vi "test bindata forth and back v2.vi"() -> ()   [LabVIEW 2018, in "LV-Julia_ZMQ-Roundtrip_lib.lvlib"]
uses:
  LV-Julia_ZMQ-Roundtrip_lib.lvlib
  05036e79-a137-49d8-b8bd-98c2707dfc19.vi
  d20d9b8d-18a0-4bcc-837d-245d5138e077.vi
  42358c4e-b4d2-4416-9aa8-9e7cd75d6887.vi
  32c35eaf-297e-4906-af2c-c0a637e2c9ed.vi
  05036e79-a137-49d8-b8bd-98c2707dfc19.vi/b16ececd-46f8-40b8-a446-7cfb86b2ab33.vi
  05036e79-a137-49d8-b8bd-98c2707dfc19.vi/2e3b4c87-8736-4d5a-badb-c1f06a639308.vi
  05036e79-a137-49d8-b8bd-98c2707dfc19.vi/c6e5ccd4-8fd0-42b7-a10f-f76efdbd56f8.vi
  05036e79-a137-49d8-b8bd-98c2707dfc19.vi/4bd48677-245d-4e5f-868b-8f16d0eed5f9.vi
  d20d9b8d-18a0-4bcc-837d-245d5138e077.vi/f1c83453-ef33-4fe1-b386-67f83703432c.vi
  d20d9b8d-18a0-4bcc-837d-245d5138e077.vi/8a46b226-3b99-41cc-8c76-34d3a32b2277.vi
  d20d9b8d-18a0-4bcc-837d-245d5138e077.vi/43989767-5720-44c7-93b6-0b6a2919d7cf.vi
  d20d9b8d-18a0-4bcc-837d-245d5138e077.vi/9fed65f7-bb03-4c69-9a7f-41e28756e77e.vi
  42358c4e-b4d2-4416-9aa8-9e7cd75d6887.vi/cf6770c6-5421-4e55-ac7c-041de9712558.vi
  32c35eaf-297e-4906-af2c-c0a637e2c9ed.vi/188cd67f-af9e-4385-87fc-606998336bf3.vi
  05036e79-a137-49d8-b8bd-98c2707dfc19.vi/2e3b4c87-8736-4d5a-badb-c1f06a639308.vi/0d828339-51f4-44c0-8bf4-a630556f2914.vi
  05036e79-a137-49d8-b8bd-98c2707dfc19.vi/c6e5ccd4-8fd0-42b7-a10f-f76efdbd56f8.vi/48ec535c-94cf-46ee-ad69-877121677c8d.vi
  05036e79-a137-49d8-b8bd-98c2707dfc19.vi/4bd48677-245d-4e5f-868b-8f16d0eed5f9.vi/cfc365a5-ff30-4df4-9512-66e4ce510117.vi
  d20d9b8d-18a0-4bcc-837d-245d5138e077.vi/8a46b226-3b99-41cc-8c76-34d3a32b2277.vi/842278c5-22e2-4c5f-9198-1cb88e2c7913.vi
  d20d9b8d-18a0-4bcc-837d-245d5138e077.vi/43989767-5720-44c7-93b6-0b6a2919d7cf.vi/3fbea689-4e70-446c-941a-28847dd52786.vi
  d20d9b8d-18a0-4bcc-837d-245d5138e077.vi/9fed65f7-bb03-4c69-9a7f-41e28756e77e.vi/d06b43ce-1229-4c8e-ae12-06e360d86b4b.vi
  42358c4e-b4d2-4416-9aa8-9e7cd75d6887.vi/cf6770c6-5421-4e55-ac7c-041de9712558.vi/ff975c95-9218-4502-b1fb-c3afa3f1137a.vi
  42358c4e-b4d2-4416-9aa8-9e7cd75d6887.vi/cf6770c6-5421-4e55-ac7c-041de9712558.vi/8deb10bf-3ab6-43d7-9d03-a9f5031347ae.vi
  32c35eaf-297e-4906-af2c-c0a637e2c9ed.vi/188cd67f-af9e-4385-87fc-606998336bf3.vi/2fc9f105-f463-40b6-badf-6ec593535007.vi
  32c35eaf-297e-4906-af2c-c0a637e2c9ed.vi/188cd67f-af9e-4385-87fc-606998336bf3.vi/ec56ee5c-7c2f-43e7-af84-ae094accc5e5.vi
  05036e79-a137-49d8-b8bd-98c2707dfc19.vi/2e3b4c87-8736-4d5a-badb-c1f06a639308.vi/0d828339-51f4-44c0-8bf4-a630556f2914.vi/dacc63a1-9bba-4eb3-b6b7-9f46c6cc7eba.vi
  05036e79-a137-49d8-b8bd-98c2707dfc19.vi/c6e5ccd4-8fd0-42b7-a10f-f76efdbd56f8.vi/48ec535c-94cf-46ee-ad69-877121677c8d.vi/1c39fd07-564b-4c6f-bc60-59ab712499e7.vi
  05036e79-a137-49d8-b8bd-98c2707dfc19.vi/4bd48677-245d-4e5f-868b-8f16d0eed5f9.vi/cfc365a5-ff30-4df4-9512-66e4ce510117.vi/5adf2ae5-6315-4e22-a618-f07e80211284.vi
  d20d9b8d-18a0-4bcc-837d-245d5138e077.vi/8a46b226-3b99-41cc-8c76-34d3a32b2277.vi/842278c5-22e2-4c5f-9198-1cb88e2c7913.vi/7c3e2bfc-f57e-4656-b3d7-5471c41a7a80.vi
  d20d9b8d-18a0-4bcc-837d-245d5138e077.vi/43989767-5720-44c7-93b6-0b6a2919d7cf.vi/3fbea689-4e70-446c-941a-28847dd52786.vi/ba37dff2-851a-4f27-b061-35721d4f87d2.vi
  d20d9b8d-18a0-4bcc-837d-245d5138e077.vi/9fed65f7-bb03-4c69-9a7f-41e28756e77e.vi/d06b43ce-1229-4c8e-ae12-06e360d86b4b.vi/81e6b4db-f1ca-4562-b9cd-32ce0e0334a5.vi
  05036e79-a137-49d8-b8bd-98c2707dfc19.vi/2e3b4c87-8736-4d5a-badb-c1f06a639308.vi/0d828339-51f4-44c0-8bf4-a630556f2914.vi/dacc63a1-9bba-4eb3-b6b7-9f46c6cc7eba.vi/dc3be9b1-6013-443b-b0cf-b3c472992a41.vi
  05036e79-a137-49d8-b8bd-98c2707dfc19.vi/c6e5ccd4-8fd0-42b7-a10f-f76efdbd56f8.vi/48ec535c-94cf-46ee-ad69-877121677c8d.vi/1c39fd07-564b-4c6f-bc60-59ab712499e7.vi/3418dce5-cf0d-4204-8015-2e708795db54.vi
  05036e79-a137-49d8-b8bd-98c2707dfc19.vi/4bd48677-245d-4e5f-868b-8f16d0eed5f9.vi/cfc365a5-ff30-4df4-9512-66e4ce510117.vi/5adf2ae5-6315-4e22-a618-f07e80211284.vi/54620dc9-9476-40af-bea6-8759de6f1d7f.vi
  d20d9b8d-18a0-4bcc-837d-245d5138e077.vi/8a46b226-3b99-41cc-8c76-34d3a32b2277.vi/842278c5-22e2-4c5f-9198-1cb88e2c7913.vi/7c3e2bfc-f57e-4656-b3d7-5471c41a7a80.vi/5dbab519-c520-424a-a111-2dba0746d6c9.vi
  d20d9b8d-18a0-4bcc-837d-245d5138e077.vi/43989767-5720-44c7-93b6-0b6a2919d7cf.vi/3fbea689-4e70-446c-941a-28847dd52786.vi/ba37dff2-851a-4f27-b061-35721d4f87d2.vi/1f70fe1b-f6c9-4ec3-89a2-80c2ccc4b870.vi
  d20d9b8d-18a0-4bcc-837d-245d5138e077.vi/9fed65f7-bb03-4c69-9a7f-41e28756e77e.vi/d06b43ce-1229-4c8e-ae12-06e360d86b4b.vi/81e6b4db-f1ca-4562-b9cd-32ce0e0334a5.vi/f5ddac4b-e08c-43f1-8e9c-0831b4c04b92.vi
  check ID validity.vi
  bindata subset by kwarg_name.vi
  <vilib>/Utility/error.llb/Error Cluster From Error Code.vi
panel:
  out "error out 2":errorcluster
  out "error out":errorcluster
  out "out 3D 2":dbl[][][](array[numeric]) format="%.2f"
  out "out 2D 2":dbl[][](array[numeric]) format="%.2f"
  out "out 1D 2":dbl[](array[numeric]) format="%.2f"
  in  "dims0":u8=2 min=1 max=3
  in  "type0":i64
  out "sent 3D":dbl[][][](array[numeric])
  out "sent 2D":dbl[][](array[numeric])
  out "sent 1D":dbl[](array[numeric])
  out "out 1D":i64[](array[numeric])
  out "out 2D":i64[][](array[numeric])
  out "out 3D":i64[][][](array[numeric])
  in  "type1":dbl
  in  "dims1":u8=2 min=1 max=3
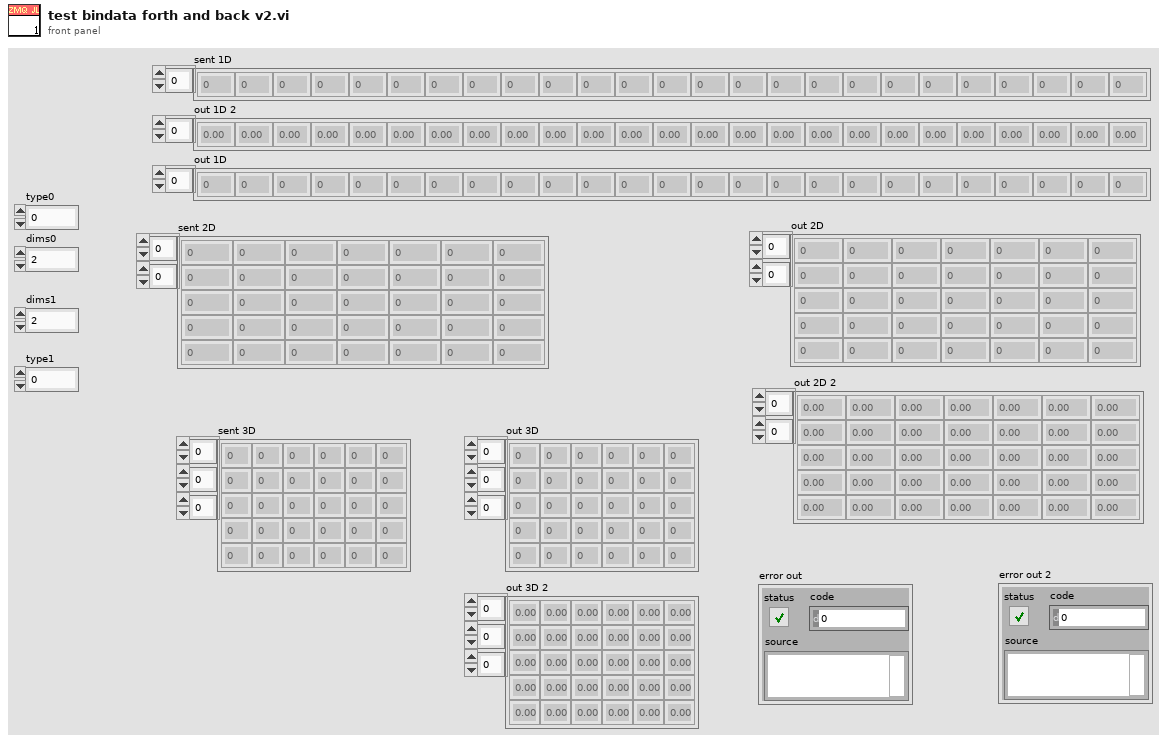
[diagram p1: front panel]
types:
  T1 = typedef "Bindata&description.ctl" = cluster{"bindata_descr":T2[], "bindata":u8[]}
  T2 = typedef "LV-Julia_ZMQ-Roundtrip_lib.lvlib/Bindata description.ctl" = cluster{"nofbytes":i32, "numtype":string, "start":i32, "arrdims":i32[], "kwarg_name":string, "category":string}
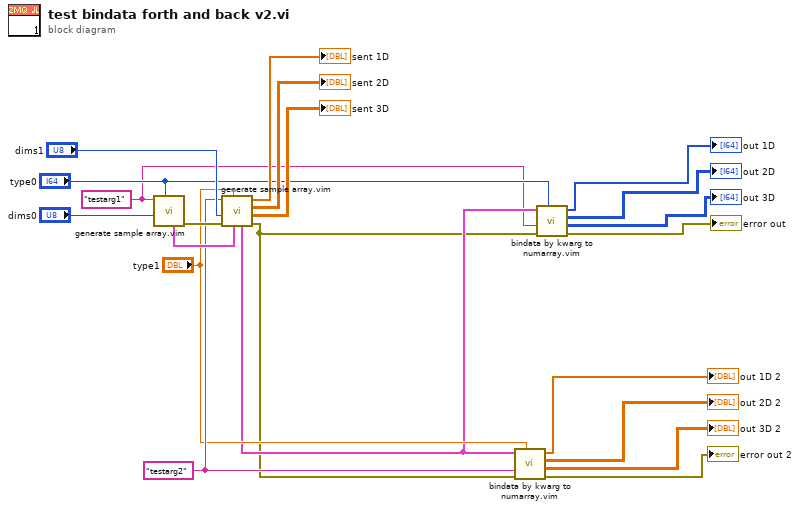
[diagram p0: block diagram]
diagram:
  w1 = "testarg1" ("kwarg_name")
  w10 = "testarg2" ("kwarg_name")
  n1 = call "generate sample array.vim"("type"="type0", "dims"="dims0", "kwarg_name"=w1) -> ("error out"=w16:errorcluster, "Bindata & descr out"=w17:T1)  [unwired: 3 in, 4 out]
  n2 = call "generate sample array.vim"("Bindata & descr in"=w17, "type"="type1", "error in (no error)"=w16, "dims"="dims1", "kwarg_name"=w10) -> ("error out"=w2:errorcluster, "Array 3D"=→"sent 3D":dbl[][][], "Array 2D"=→"sent 2D":dbl[][], "Array 1D"=→"sent 1D":dbl[], "Bindata & descr out"=w3:T1)  [unwired: 1 in, 1 out]
  n3 = call "bindata by kwarg to numarray.vim"("type in"="type1", "error in (no error)"=w2, "kwarg_name"=w10, "Bindata & descr in"=w3) -> ("error out"=→"error out 2":errorcluster, "numarray 3D"=→"out 3D 2":dbl[][][], "numarray 2D"=→"out 2D 2":dbl[][], "numarray 1D"=→"out 1D 2":dbl[])  [unwired: 4 in]
  n4 = call "bindata by kwarg to numarray.vim"("type in"="type0", "error in (no error)"=w2, "kwarg_name"=w1, "Bindata & descr in"=w3) -> ("error out"=→"error out":errorcluster, "numarray 3D"=→"out 3D":i64[][][], "numarray 2D"=→"out 2D":i64[][], "numarray 1D"=→"out 1D":i64[])  [unwired: 4 in]
